vi "channeldata_2ch_complex.vi"() -> ()   [LabVIEW 2019]
panel:
  out "Error Out":errorcluster
  in  "TDMS File":path=path "C:/Python/projects/nitdms/tests/tdms_files/channeldata_2ch_complex.tdms"
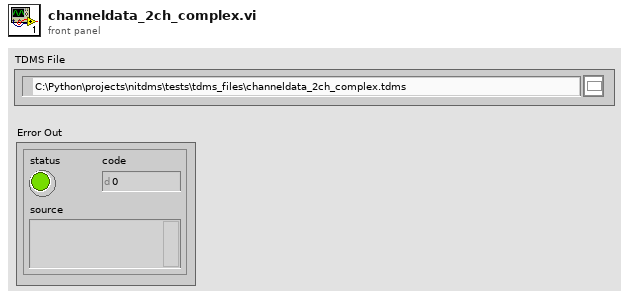
[diagram p1: front panel]
types:
  T1 = enum16{"open", "open or create", "create or replace", "create", "open (read-only)"}
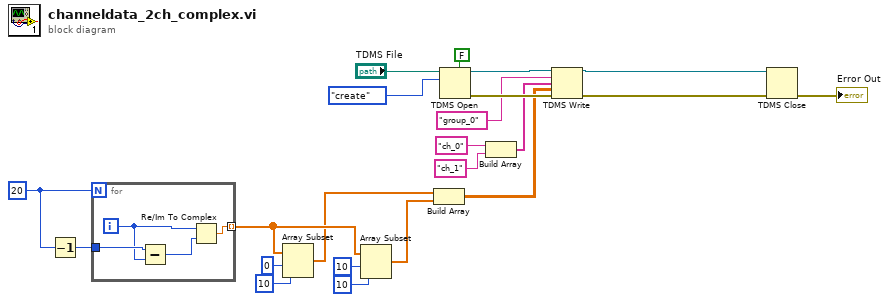
[diagram p0: block diagram]
diagram:
  w3 = 20
  n1 = Decrement(x=w3) -> (x-1=w2:i32)
  n2 = for {
    N: w3 -> [_]
    tunnel: [w23] -> w11 mode=indexing
    tunnel: w2 -> [w26]
    i -> [w25]
    n3 = Subtract(x=w26, y=w25) -> (x-y=w24:i32)
    n4 = Re/Im To Complex(1:w24, 2:w25) -> (0:w23:cdb)
  }
  n5 = Array Subset(array=w11, index=0, length=10) -> (w10:cdb[])
  n6 = Array Subset(array=w11, index=10, length=10) -> (w9:cdb[])
  n7 = Build Array(w10, w9) -> (w1:cdb[][])
  n8 = TDMS Open(5:FALSE ("create index file? (T)"), 10:T1."create" ("operation (0:open)"), 11:"TDMS File") -> (0:w18:errorcluster, 3:w17:refnum<k34>)  [unwired: 4 in]
  n9 = Build Array("ch_0", "ch_1") -> (w6:string[])
  n10 = TDMS Write(0:w17, 5:"group_0", 7:w6, 9:w1, 11:w18) -> (4:w4:refnum<k34>, 15:w5:errorcluster)  [unwired: 1 in, 2 out]
  n11 = TDMS Close(8:w5, 11:w4) -> (0:→"Error Out":errorcluster)  [unwired: 1 out]
